vi "add.vi"(8 "error in (no error)":errorcluster, 11 "classB in":refnum<class "classB.lvclass">) -> (0 "error out":errorcluster, 2 "String":string, 3 "classB out":refnum<class "classB.lvclass">)   [LabVIEW 2020, in "classB.lvclass"]
uses:
  classB.lvclass
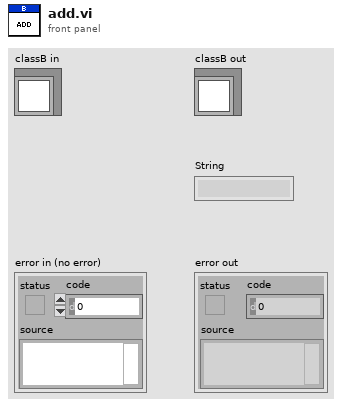
[diagram p1: front panel]
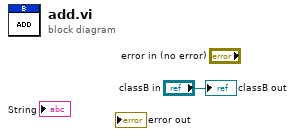
[diagram p0: block diagram]
diagram:
  "classB out" <- "classB in"
